vi "Configure Generator External Attenuation.vi"(8 "error in (no error)":errorcluster, 9 "External Attenuation (0.0)":dbl format="%^.3e", 10 "Instance (1)":i32=1, 11 "VISA resource name":refnum<visa-resource-name>) -> (0 "error out":errorcluster, 3 "VISA resource name out":refnum<visa-resource-name>)   [LabVIEW 2015, in "Rohde&Schwarz CMXP GPRF.lvlib"]
doc: "Defines an external attenuation value.\n\nAttribute:\nRSCMXPGPRF_ATTR_GENERATOR_EXTERNAL_ATTENUTATION\n\nRemote-control command:\nSOURce:GPRF:GEN<i>:RFSettings:EATTenuation"
uses:
  <instrlib>/Rohde&Schwarz CMXP GPRF/Rohde&Schwarz CMXP GPRF.lvlib
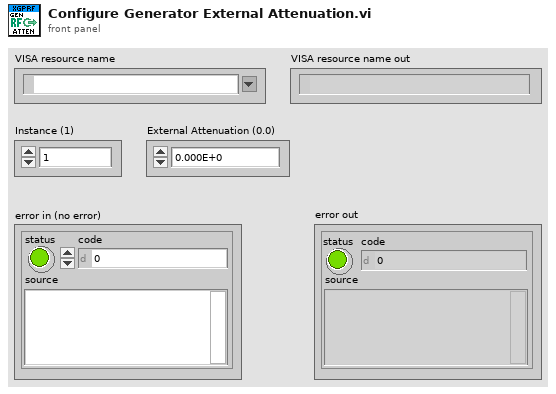
[diagram p1: front panel]
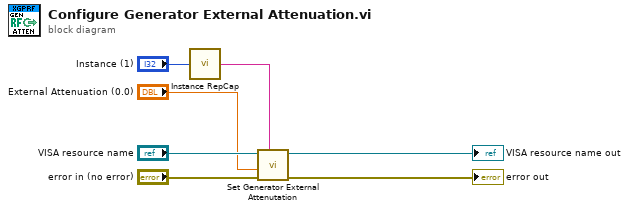
[diagram p0: block diagram]
diagram:
  n1 = call <instrlib>:"Instance RepCap.vi"("instance  in"="Instance (1)") -> ("instance out"=w6:string)
  n2 = call "Set Generator External Attenutation"("Repeated Capabilities"=w6, "error in (no error)"="error in (no error)", "Generator External Attenutation (0.0)"="External Attenuation (0.0)", "instrument handle"="VISA resource name") -> ("error out"=→"error out":errorcluster, "instrument handle out"=→"VISA resource name out":refnum<visa-resource-name>)  [unwired: 6 in]
